vi "DAQ_Volt_Measure.vi"   [LabVIEW 2025]
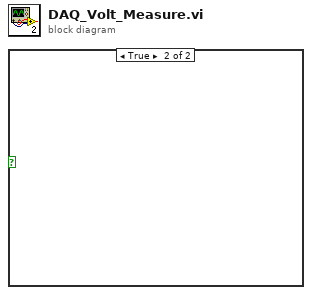
[diagram p0: block diagram]
diagram:
  n1 = case shown="True" {
    selector: _ -> [_ _]
    frame False {
    }
    frame True {
    }
  }
